vi "DataLog Aggregation Recovery Master.vi"(11 "error in (no error)":errorcluster) -> (15 "error out":errorcluster)   [LabVIEW 2012]
doc: "This VI handles the recovery of the recovery file and the flushing of its contents to the tag logs. The data structure of the aggregation buffer is designed to allow quick updates of the recovery file. This is at odds with easy recovery. Consequently, the recovery operation is somewhat involved.\n\nIn order to perform the recovery, this VI requires that the related MCVD global variables be initialized as before the crash. All data up to the last recovery file update is retrieved and written to the various tag logs. The delay between recovery file updates therefore limits the amount of data loss."
uses:
  typedefs/t_DataLog Tag Hash Methods.ctl
  glb_DataLog Runtime Parameterisation.vi
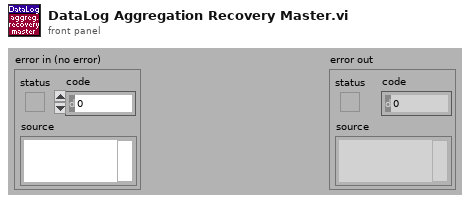
[diagram p1: front panel]
types:
  T1 = typedef "t_DataLog Tag Hash Methods.ctl" = enum16{"initialize", "add tag", "index tag", "lookup", "#tags", "cleanup", "write recovery", "read recovery", "delete recovery"}
  T2 = typedef "t_DataLog Aggregation Entry.ctl" = cluster{"tag index":i32, "point":T3}
  T3 = typedef "t_DataLog Point.ctl" = cluster{"time":dbl, "value":dbl}
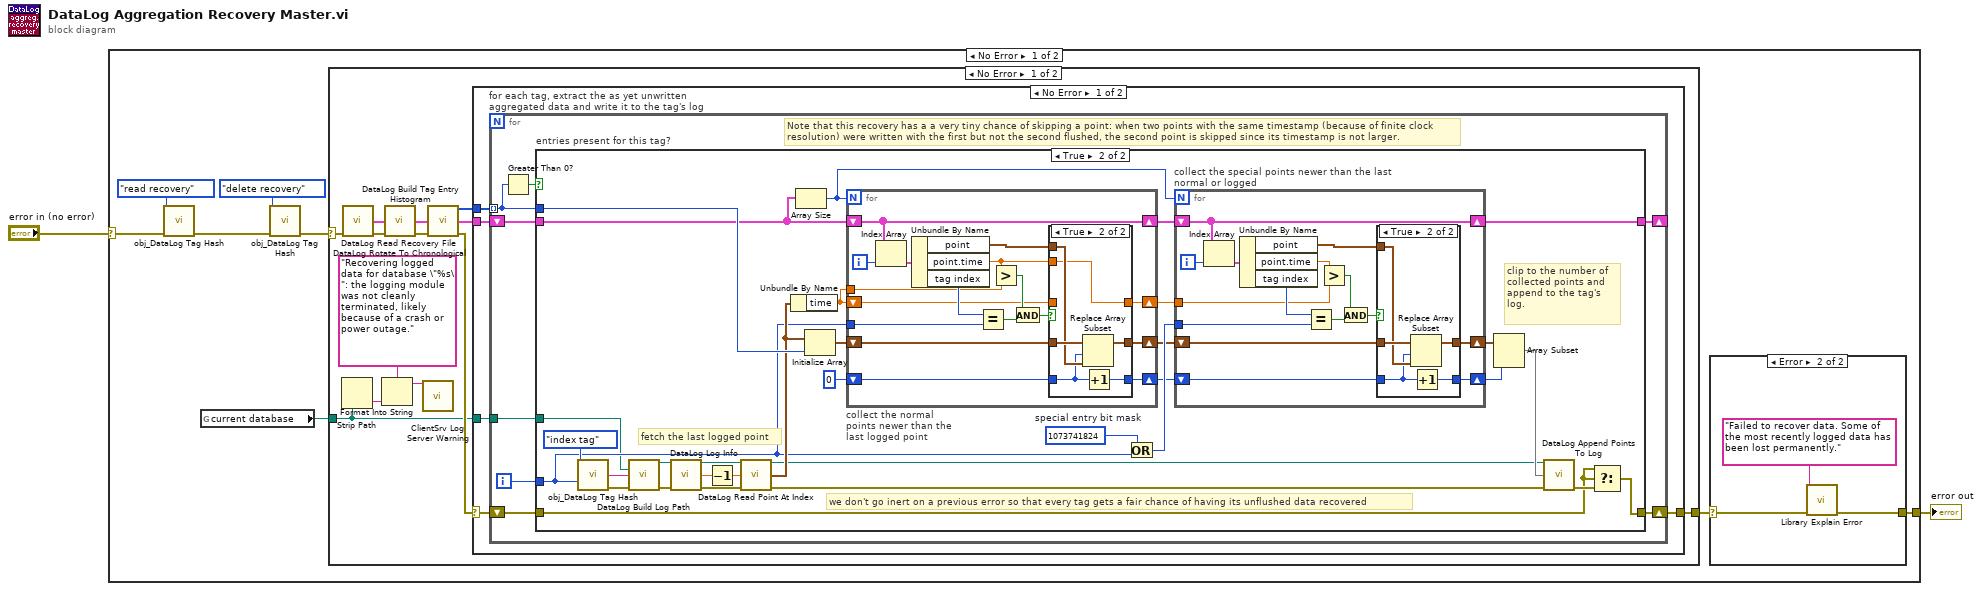
[diagram p0: block diagram]
diagram:
  n1 = case shown="No Error" "error in (no error)" {
    selector: "error in (no error)" -> [w7 w125]
    tunnel: [w8 w125] -> w1
    frame No Error {
      n2 = call "obj_DataLog Tag Hash.vi"("method"=t_DataLog_Tag_Hash_Methods."read recovery", "error in (no error)"=w7) -> ("error out"=w5:errorcluster)  [unwired: 10 in, 3 out]
      n3 = global read "glb_DataLog Runtime Parameterisation.vi" "current database"() -> (w3:path)
      n4 = call "obj_DataLog Tag Hash.vi"("method"=t_DataLog_Tag_Hash_Methods."delete recovery", "error in (no error)"=w5) -> ("error out"=w4:errorcluster)  [unwired: 10 in, 3 out]
      n5 = case shown="No Error" w4 {
        selector: w4 -> [w19 _]
        tunnel: [w20 _] -> w9
        tunnel: w3 -> [w16 _]
        frame No Error {
          n6 = Strip Path(path=w16) -> (name=w17:string)  [unwired: 1 out]
          n7 = call "DataLog Read Recovery File.vi"("error in (no error)"=w19) -> ("aggregation entries"=w26:T2[], "error out"=w27:errorcluster)  [unwired: 13 in]
          n8 = Format Into String(format string="Recovering logged data for database \"%s\": the logging module was not cleanly terminated, likely because of a crash or power outage." ("message (use cluster)"), w17) -> (resulting string=w15:string)  [unwired: 2 in, 1 out]
          n9 = call "DataLog Rotate To Chronological.vi"("aggregation entries in"=w26, "error in (no error)"=w27) -> ("aggregation entries out"=w25:T2[], "dup error"=w24:errorcluster)  [unwired: 12 in]
          n10 = call "ClientSrv Log Server Warning.vi"("message (use cluster)"=w15) -> ()  [unwired: 15 in]
          n11 = call "DataLog Build Tag Entry Histogram.vi"("aggregation entries in"=w25, "error in (no error)"=w24) -> ("entries per tag"=w23:i32[], "aggregation entries out"=w22:T2[], "dup error"=w21:errorcluster)  [unwired: 11 in]
          n12 = case shown="No Error" w21 {
            selector: w21 -> [w30 w124]
            tunnel: w23 -> [w32 _]
            tunnel: w22 -> [w31 _]
            tunnel: [w29 w124] -> w20
            tunnel: w16 -> [w28 _]
            frame No Error {
              n13 = for "for each tag, extract the as yet unwritten aggregated data and write it to the tag's log" {
                tunnel: w32 -> [w37] mode=indexing
                shift-right: [w38] -> _
                shift-left: w31 -> [w39]
                shift-right: [w36] -> w29
                shift-left: w30 -> [w34]
                tunnel: w28 -> [w33]
                i -> [w35]
                # "Note that this recovery has a a very tiny chance of skipping a point: when two points with the same timestamp (because of finite clock resolution) were written with the first but not the second flushed, the second point is skipped since its timestamp is not larger."
                n14 = Greater Than 0?(x=w37) -> (x > 0?=w40:bool)
                n15 = case "entries present for this tag?" shown="True" w40 {
                  tunnel: w39 -> [w42 w73]
                  tunnel: [w42 w64] -> w38
                  tunnel: w37 -> [_ w75]
                  tunnel: w34 -> [w41 w57]
                  tunnel: [w41 w59] -> w36
                  tunnel: w35 -> [_ w44]
                  tunnel: w33 -> [_ w43]
                  frame False {
                  }
                  frame True {
                    w69 = 1073741824  # special entry bit mask
                    # "fetch the last logged point"
                    # "clip to the number of\ncollected points and\nappend to the tag's\nlog."
                    # "we don't go inert on a previous error so that every tag gets a fair chance of having its unflushed data recovered"
                    n16 = call "obj_DataLog Tag Hash.vi"("method"=t_DataLog_Tag_Hash_Methods."index tag", "tag index in"=w44) -> ("tag out"=w47:string, "error out"=w46:errorcluster)  [unwired: 10 in, 2 out]
                    n17 = call "DataLog Build Log Path.vi"("database path"=w43, "tag"=w47, "error in (no error)"=w46) -> ("tag log directory"=w48:path, "error out"=w49:errorcluster)  [unwired: 11 in]
                    n18 = call "DataLog Log Info.vi"("tag log directory"=w48, "error in (no error)"=w49) -> ("dup tag log directory"=w55:path, "size"=w53:dbl, "error out"=w56:errorcluster)  [unwired: 10 in, 1 out]
                    n19 = Decrement(x=w53) -> (x-1=w54:dbl)
                    n20 = call "DataLog Read Point At Index.vi"("tag log directory"=w55, "log index"=w54, "error in (no error)"=w56) -> ("dup tag log directory"=w50:path, "point"=w51:T3, "error out"=w52:errorcluster)  [unwired: 10 in]
                    n21 = Unbundle By Name(w51) -> ("time"=w71:dbl)
                    n22 = Array Size(array=w73) -> (size(s)=w60:i32)
                    n23 = Initialize Array(w51, w75) -> (w74:T3[])
                    n24 = for "collect the normal points newer than the last logged point" {
                      N: w60 -> [_]
                      shift-right: [w105] -> w66
                      shift-left: w74 -> [w109]
                      shift-right: [w114] -> w65
                      shift-left: w73 -> [w114]
                      shift-right: [w106] -> w67
                      shift-left: 0 -> [w107]
                      tunnel: w44 -> [w111]
                      shift-right: [w101] -> w70
                      shift-left: w71 -> [w99]
                      tunnel: w71 -> [w98]
                      i -> [w113]
                      n25 = Index Array(array=w114, index=w113) -> (element=w112:T2)
                      n26 = Unbundle By Name(w112) -> ("point"=w108:T3, "point.time"=w100:dbl, "tag index"=w110:i32)
                      n27 = Equal?(x=w110, y=w111) -> (x = y?=w102:bool)
                      n28 = Greater?(x=w100, y=w98) -> (0:w103:bool)
                      n29 = And(x=w103, y=w102) -> (x .and. y?=w104:bool)
                      n30 = case shown="True" w104 {
                        tunnel: w109 -> [w116 w123]
                        tunnel: w108 -> [_ w122]
                        tunnel: w107 -> [w117 w121]
                        tunnel: [w117 w120] -> w106
                        tunnel: [w116 w119] -> w105
                        tunnel: [w115 w118] -> w101
                        tunnel: w99 -> [w115 _]
                        tunnel: w100 -> [_ w118]
                        frame False {
                        }
                        frame True {
                          n31 = Replace Array Subset(array=w123, new element=w122, index=w121) -> (w119:T3[])
                          n32 = Increment(x=w121) -> (x+1=w120:i32)
                        }
                      }
                    }
                    n33 = Or(x=w69, y=w44) -> (x .or. y?=w68:i32)
                    n34 = for "collect the special points newer than the last normal or logged" {
                      N: w60 -> [_]
                      shift-right: [w81] -> w63
                      shift-left: w66 -> [w85]
                      shift-right: [w90] -> w64
                      shift-left: w65 -> [w90]
                      shift-right: [w82] -> w62
                      shift-left: w67 -> [w83]
                      tunnel: w68 -> [w87]
                      tunnel: w70 -> [w77]
                      i -> [w89]
                      n35 = Index Array(array=w90, index=w89) -> (element=w88:T2)
                      n36 = Unbundle By Name(w88) -> ("point"=w84:T3, "point.time"=w76:dbl, "tag index"=w86:i32)
                      n37 = Equal?(x=w86, y=w87) -> (x = y?=w78:bool)
                      n38 = Greater?(x=w76, y=w77) -> (0:w79:bool)
                      n39 = And(x=w79, y=w78) -> (x .and. y?=w80:bool)
                      n40 = case shown="True" w80 {
                        tunnel: w85 -> [w91 w97]
                        tunnel: w84 -> [_ w96]
                        tunnel: w83 -> [w92 w95]
                        tunnel: [w92 w94] -> w82
                        tunnel: [w91 w93] -> w81
                        frame False {
                        }
                        frame True {
                          n41 = Replace Array Subset(array=w97, new element=w96, index=w95) -> (w93:T3[])
                          n42 = Increment(x=w95) -> (x+1=w94:i32)
                        }
                      }
                    }
                    n43 = Array Subset(array=w63, length=w62) -> (w61:T3[])  [unwired: 1 in]
                    n44 = call "DataLog Append Points To Log.vi"("tag log directory"=w50, "points"=w61, "error in (no error)"=w52) -> ("error out"=w58:errorcluster)  [unwired: 11 in, 1 out]
                    n45 = Select(t=w57, s=w57, f=w58) -> (s? t:f=w59:errorcluster)
                  }
                }
              }
            }
            frame Error {
            }
          }
        }
        frame Error {
          # "When there is no hash file, there is nothing to recover.\nWhen the hash file cannot be read, we cannot recover."
        }
      }
      n46 = case shown="Error" w9 {
        selector: w9 -> [w11 w12]
        tunnel: [w11 w14] -> w8
        frame No Error {
        }
        frame Error {
          n47 = call "Library Explain Error.vi"("explanation prefix (none)"="Failed to recover data. Some of the most recently logged data has been lost permanently." ("string"), "error in (no error)"=w12) -> ("explained error"=w14:errorcluster)  [unwired: 13 in]
        }
      }
    }
    frame Error {
    }
  }
  "error out" <- w1
